vi "Eurotherm - Front Panel.vi"() -> ()   [LabVIEW 2011]
uses:
  Common/Utilities/VI Control/Control - Display State.ctl
panel:
  in  "Setup":bool
  out "Activity":bool
  out "Numeric":i32
  in  "stop":bool
  in  "Tab Control":T1(tab)
  in  "Set Point Read":dbl format="%.3f"
  in  "Ramp Rate 1":dbl format="%.3f"
  in  "Type 1":u16(ring) items=["Step", "Ramp"]
  in  "Clear Graph 1":bool
  in  "AutoTune 1":bool
  out "XY Graph 1":cluster{"Data":cluster{"Time":dbl, "Y":dbl}[]}[](graph)
  out "Temp 1":dbl format="%.3f"
  out "Heater Output 1":dbl format="%.3f"
  in  "Max Output 1":dbl format="%.3f"
  in  "D 1":dbl format="%.3f"
  in  "I 1":dbl format="%.3f"
  in  "P 1":dbl format="%.3f"
  in  "Set Point 1":dbl min=0.0 max=40.0 format="%.3f"
  in  "Set Point Read 2":dbl format="%.3f"
  in  "P 2":dbl format="%.3f"
  in  "I 2":dbl format="%.3f"
  in  "D 2":dbl format="%.3f"
  out "Temp 2":dbl format="%.3f"
  out "Heater Output 2":dbl format="%.3f"
  in  "Set Point 2":dbl min=0.0 max=40.0 format="%.3f"
  in  "Max Output 2":dbl format="%.3f"
  out "XY Graph 2":cluster{"Data":cluster{"Time":dbl, "Y":dbl}[]}[](graph)
  in  "AutoTune 2":bool
  in  "Clear Graph 2":bool
  in  "Type 2":u16(ring) items=["Step", "Ramp"]
  in  "Ramp Rate 2":dbl format="%.3f"
  in  "P 3":dbl format="%.3f"
  in  "I 3":dbl format="%.3f"
  in  "D 3":dbl format="%.3f"
  out "Temp 3":dbl format="%.3f"
  out "Heater Output 3":dbl format="%.3f"
  in  "Set Point 3":dbl min=0.0 max=100.0 format="%.3f"
  in  "Max Output 3":dbl format="%.3f"
  out "XY Graph 3":cluster{"Data":cluster{"Time":dbl, "Y":dbl}[]}[](graph)
  in  "AutoTune 3":bool
  in  "Clear Graph 3":bool
  in  "Type 3":u16(ring) items=["Step", "Ramp"]
  in  "Ramp Rate 3":dbl format="%.3f"
  in  "Set Point Read 3":dbl format="%.3f"
  in  "P 4":dbl format="%.3f"
  in  "I 4":dbl format="%.3f"
  in  "D 4":dbl format="%.3f"
  out "Temp 4":dbl format="%.3f"
  out "Heater Output 4":dbl format="%.3f"
  in  "Set Point 4":dbl min=0.0 max=100.0 format="%.3f"
  in  "Max Output 4":dbl format="%.3f"
  out "XY Graph 4":cluster{"Data":cluster{"Time":dbl, "Y":dbl}[]}[](graph)
  in  "AutoTune 4":bool
  in  "Clear Graph 4":bool
  in  "Type 4":u16(ring) items=["Step", "Ramp"]
  in  "Ramp Rate 4":dbl format="%.3f"
  in  "Set Point Read 4":dbl format="%.3f"
  in  "P 5":dbl format="%.3f"
  in  "I 5":dbl format="%.3f"
  in  "D 5":dbl format="%.3f"
  out "Temp 5":dbl format="%.3f"
  out "Heater Output 5":dbl format="%.3f"
  in  "Set Point 5":dbl min=0.0 max=100.0 format="%.3f"
  in  "Max Output 5":dbl format="%.3f"
  out "XY Graph 5":cluster{"Data":cluster{"Time":dbl, "Y":dbl}[]}[](graph)
  in  "AutoTune 5":bool
  in  "Clear Graph 5":bool
  in  "Type 5":u16(ring) items=["Step", "Ramp"]
  in  "Ramp Rate 5":dbl format="%.3f"
  in  "Set Point Read 5":dbl format="%.3f"
  in  "P 6":dbl format="%.3f"
  in  "I 6":dbl format="%.3f"
  in  "D 6":dbl format="%.3f"
  out "Temp 6":dbl format="%.3f"
  out "Heater Output 6":dbl format="%.3f"
  in  "Set Point 6":dbl min=0.0 max=100.0 format="%.3f"
  in  "Max Output 6":dbl format="%.3f"
  out "XY Graph 6":cluster{"Data":cluster{"Time":dbl, "Y":dbl}[]}[](graph)
  in  "AutoTune 6":bool
  in  "Clear Graph 6":bool
  in  "Type 6":u16(ring) items=["Step", "Ramp"]
  in  "Ramp Rate 6":dbl format="%.3f"
  in  "Set Point Read 6":dbl format="%.3f"
  in  "P 7":dbl format="%.3f"
  in  "I 7":dbl format="%.3f"
  in  "D 7":dbl format="%.3f"
  out "Temp 7":dbl format="%.3f"
  out "Heater Output 7":dbl format="%.3f"
  in  "Set Point 7":dbl min=0.0 max=100.0 format="%.3f"
  in  "Max Output 7":dbl format="%.3f"
  out "XY Graph 7":cluster{"Data":cluster{"Time":dbl, "Y":dbl}[]}[](graph)
  in  "AutoTune 7":bool
  in  "Clear Graph 7":bool
  in  "Type 7":u16(ring) items=["Step", "Ramp"]
  in  "Ramp Rate 7":dbl format="%.3f"
  in  "Set Point Read 7":dbl format="%.3f"
  in  "P 8":dbl format="%.3f"
  in  "I 8":dbl format="%.3f"
  in  "D 8":dbl format="%.3f"
  out "Temp 8":dbl format="%.3f"
  out "Heater Output 8":dbl format="%.3f"
  in  "Set Point 8":dbl min=0.0 max=100.0 format="%.3f"
  in  "Max Output 8":dbl format="%.3f"
  out "XY Graph 8":cluster{"Data":cluster{"Time":dbl, "Y":dbl}[]}[](graph)
  in  "AutoTune 8":bool
  in  "Clear Graph 8":bool
  in  "Type 8":u16(ring) items=["Step", "Ramp"]
  in  "Ramp Rate 8":dbl format="%.3f"
  in  "Set Point Read 8":dbl format="%.3f"
  # "Eurotherm Temperature Controller"
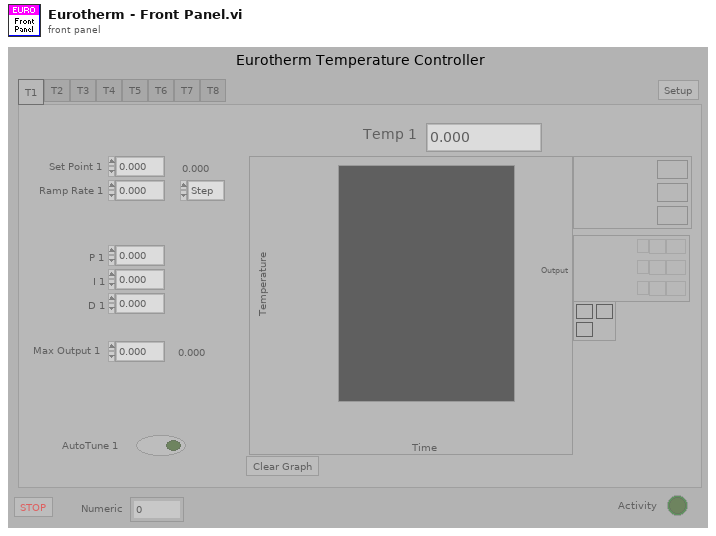
[diagram p1: front panel]
types:
  T1 = enum32{"Page 1", "Page 2", "Page 3", "Page 4", "T5", "T5 2", "T7", "T8"}
  T2 = typedef "Control - Display State.ctl" = enum16{"Enabled", "Disabled", "Disabled and Grayed"}
  T3 = enum32{"Page Enabled", "Page Disabled", "Page Disabled & Grayed"}
  T4 = cluster{"Temp 1":refnum<vi>, "Set Point 1":refnum<vi>, "P 1":refnum<vi>, "I 1":refnum<vi>, "D 1":refnum<vi>, "Heater Output 1":refnum<vi>, "Max Output 1":refnum<vi>, "XY Graph 1":refnum<vi>, "AutoTune 1":refnum<vi>, "Clear Graph 1":refnum<vi>, "Ramp Rate 1":refnum<vi>, "Type 1":refnum<vi>, "Tab Control":refnum<vi>, "Set Point Read":refnum<vi>}
  T5 = cluster{"Temp 2":refnum<vi>, "Set Point 2":refnum<vi>, "P 2":refnum<vi>, "I 2":refnum<vi>, "D 2":refnum<vi>, "Heater Output 2":refnum<vi>, "Max Output 2":refnum<vi>, "XY Graph 2":refnum<vi>, "AutoTune 2":refnum<vi>, "Clear Graph 2":refnum<vi>, "Ramp Rate 2":refnum<vi>, "Type 2":refnum<vi>, "Tab Control":refnum<vi>, "Set Point Read 2":refnum<vi>}
  T6 = cluster{"Temp 3":refnum<vi>, "Set Point 3":refnum<vi>, "P 3":refnum<vi>, "I 3":refnum<vi>, "D 3":refnum<vi>, "Heater Output 3":refnum<vi>, "Max Output 3":refnum<vi>, "XY Graph 3":refnum<vi>, "AutoTune 3":refnum<vi>, "Clear Graph 3":refnum<vi>, "Ramp Rate 3":refnum<vi>, "Type 3":refnum<vi>, "Tab Control":refnum<vi>, "Set Point Read 3":refnum<vi>}
  T7 = cluster{"Temp 4":refnum<vi>, "Set Point 4":refnum<vi>, "P 4":refnum<vi>, "I 4":refnum<vi>, "D 4":refnum<vi>, "Heater Output 4":refnum<vi>, "Max Output 4":refnum<vi>, "XY Graph 4":refnum<vi>, "AutoTune 4":refnum<vi>, "Clear Graph 4":refnum<vi>, "Ramp Rate 4":refnum<vi>, "Type 4":refnum<vi>, "Tab Control":refnum<vi>, "Set Point Read 4":refnum<vi>}
  T8 = cluster{"Temp 5":refnum<vi>, "Set Point 5":refnum<vi>, "P 5":refnum<vi>, "I 5":refnum<vi>, "D 5":refnum<vi>, "Heater Output 5":refnum<vi>, "Max Output 5":refnum<vi>, "XY Graph 5":refnum<vi>, "AutoTune 5":refnum<vi>, "Clear Graph 5":refnum<vi>, "Ramp Rate 5":refnum<vi>, "Type 5":refnum<vi>, "Tab Control":refnum<vi>, "Set Point Read 5":refnum<vi>}
  T9 = cluster{"Temp 6":refnum<vi>, "Set Point 6":refnum<vi>, "P 6":refnum<vi>, "I 6":refnum<vi>, "D 6":refnum<vi>, "Heater Output 6":refnum<vi>, "Max Output 6":refnum<vi>, "XY Graph 6":refnum<vi>, "AutoTune 6":refnum<vi>, "Clear Graph 6":refnum<vi>, "Ramp Rate 6":refnum<vi>, "Type 6":refnum<vi>, "Tab Control":refnum<vi>, "Set Point Read 6":refnum<vi>}
  T10 = cluster{"Temp 7":refnum<vi>, "Set Point 7":refnum<vi>, "P 7":refnum<vi>, "I 7":refnum<vi>, "D 7":refnum<vi>, "Heater Output 7":refnum<vi>, "Max Output 7":refnum<vi>, "XY Graph 7":refnum<vi>, "AutoTune 7":refnum<vi>, "Clear Graph 7":refnum<vi>, "Ramp Rate 7":refnum<vi>, "Type 7":refnum<vi>, "Tab Control":refnum<vi>, "Set Point Read 7":refnum<vi>}
  T11 = cluster{"Temp 8":refnum<vi>, "Set Point 8":refnum<vi>, "P 8":refnum<vi>, "I 8":refnum<vi>, "D 8":refnum<vi>, "Heater Output 8":refnum<vi>, "Max Output 8":refnum<vi>, "XY Graph 8":refnum<vi>, "AutoTune 8":refnum<vi>, "Clear Graph 8":refnum<vi>, "Ramp Rate 8":refnum<vi>, "Type 8":refnum<vi>, "Tab Control":refnum<vi>, "Set Point Read 8":refnum<vi>}
  T12 = typedef "Eurotherm - Setups.ctl" = T13[]
  T13 = typedef "Eurotherm - Setup.ctl" = cluster{"Communication":T14, "Name":string, "Enable":bool, "Max Set Point":dbl, "Min Set Point":dbl, "Units":string, "Graph Data":u32, "Sensor type":T18, "Calibration File Path":path, "Conversion Type":T19}
  T14 = typedef "Eurotherm - Communication.ctl" = cluster{"Com Port":T15, "Address":T16, "Baud Rate":T17}
  T15 = typedef "Com Port - Numeric.ctl" = i32
  T16 = typedef "Eurotherm - Address.ctl" = u8
  T17 = typedef "Com Port - Baud Rate.ctl" = u32
  T18 = typedef "Sensors - Temperature Sensor Type.ctl" = enum16{"RhFe", "Pt", "K type thermocouple", "W5 type thermocouple", "No Conversion"}
  T19 = typedef "Sensors - Conversion Type.ctl" = enum16{"Linear", "Spline"}
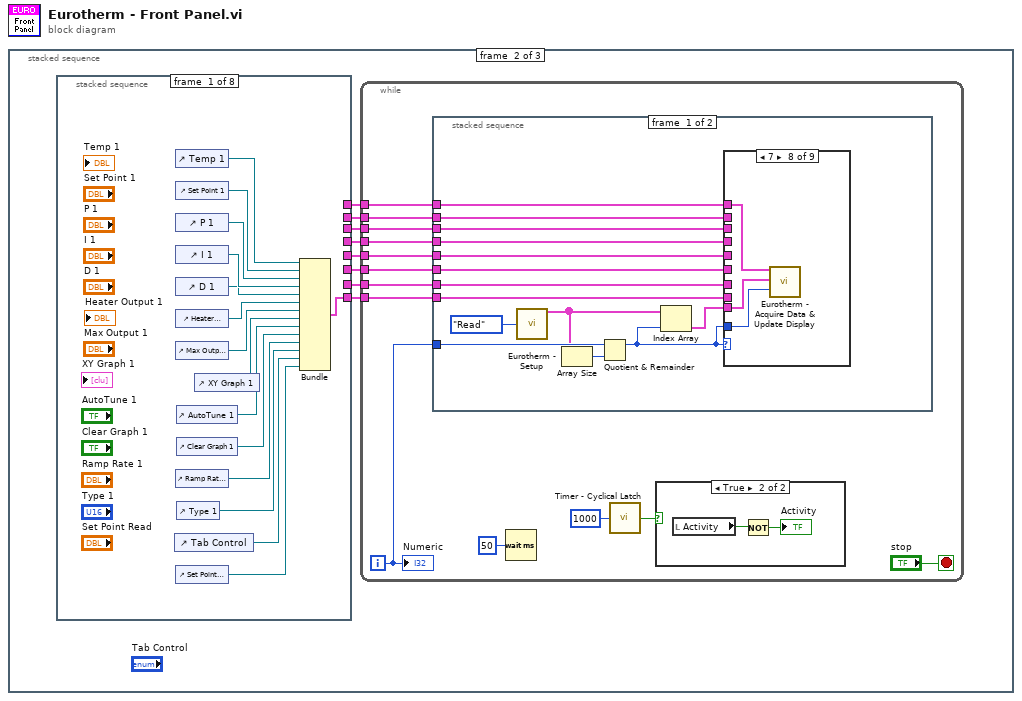
[diagram p0: block diagram]
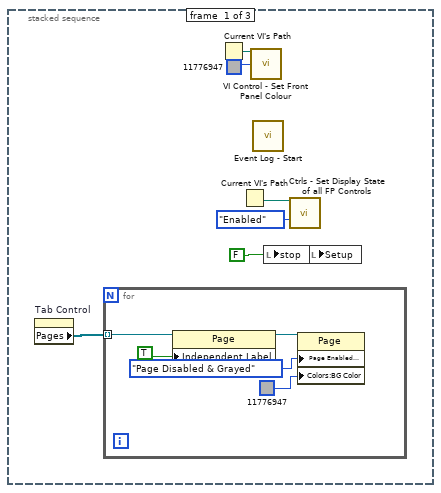
[diagram p2: hidden frame]
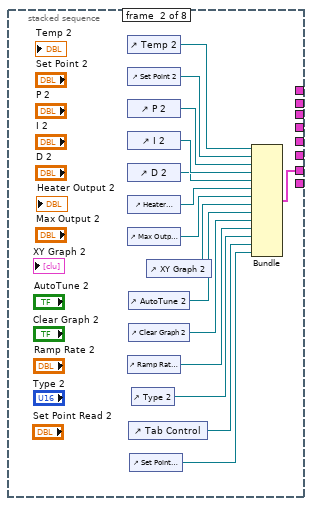
[diagram p3: hidden frame]
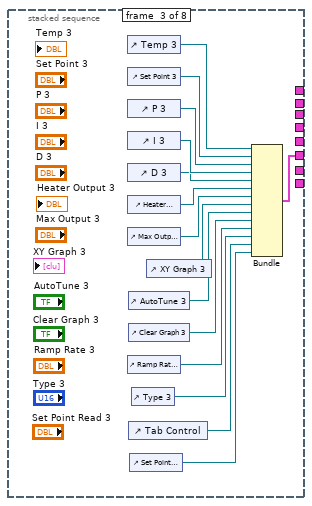
[diagram p4: hidden frame]
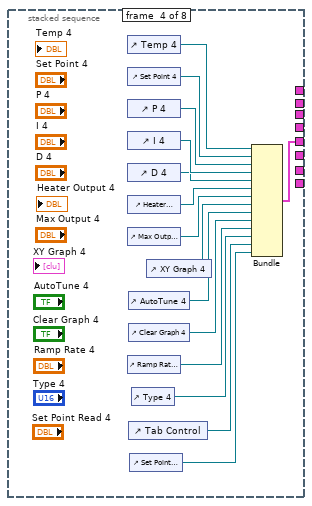
[diagram p5: hidden frame]
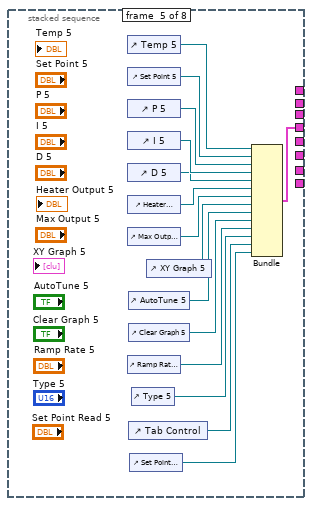
[diagram p6: hidden frame]
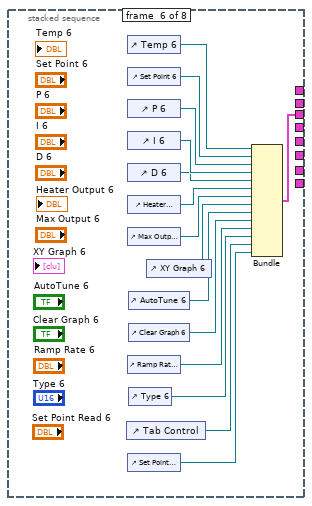
[diagram p7: hidden frame]
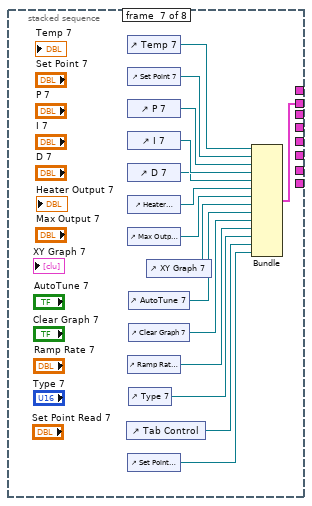
[diagram p8: hidden frame]
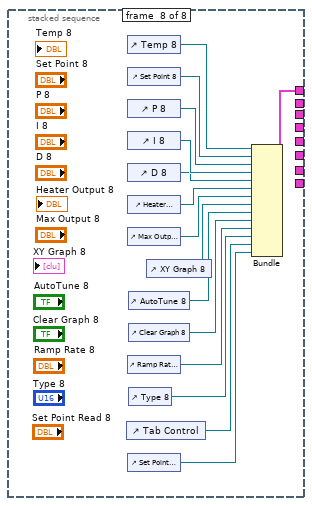
[diagram p9: hidden frame]
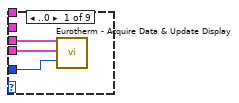
[diagram p10: hidden frame]
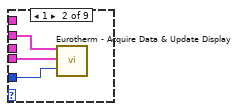
[diagram p11: hidden frame]
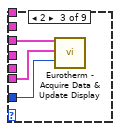
[diagram p12: hidden frame]
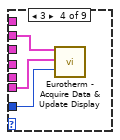
[diagram p13: hidden frame]
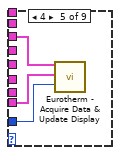
[diagram p14: hidden frame]
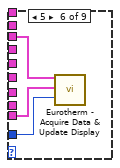
[diagram p15: hidden frame]
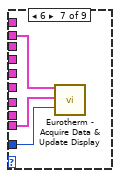
[diagram p16: hidden frame]
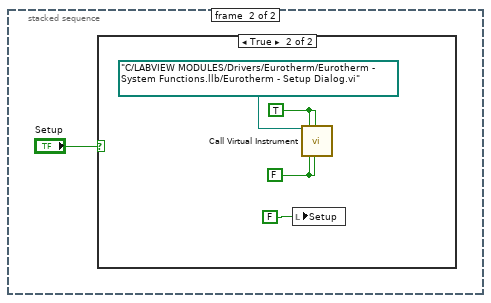
[diagram p18: hidden frame]
diagram:
  n1 = stacked-sequence {
    frame #0 {
      w1 = FALSE
      n2 = property on="Tab Control" class="TabCtl (strict)"() -> ("Pages"=w4:refnum<vi>[])  [unwired: 2 in, 2 out]
      n3 = for {
        tunnel: w4 -> [w9] mode=indexing
        n4 = property class="Page"(reference=w9, "Independent Label"=TRUE) -> (reference out=w10:refnum<vi>)  [unwired: 1 in, 1 out]
        n5 = property class="Page"(reference=w10, "Page Enabled State"=T3."Page Disabled & Grayed", "Colors:BG Color"=u32 11776947) -> ()  [unwired: 1 in, 2 out]
      }
      n6 = Current VI's Path() -> (path=w2:path)
      n7 = Current VI's Path() -> (path=w6:path)
      n8 = call "VI Control - Set Front Panel Colour.vi"("VI Path"=w2, "Front Panel Colour"=u32 11776947) -> ()  [unwired: 13 in, 1 out]
      n9 = call "Event Log - Start.vi"() -> ()  [unwired: 1 in]
      n10 = local write "stop"(w1) -> ()
      n11 = call "Ctrls - Set Display State of all FP Controls.vi"("VI Path"=w6, "Display State"=Control_-_Display_State."Enabled") -> ()  [unwired: 18 in]
      n12 = local write "Setup"(w1) -> ()
    }
    frame #1 {
      n13 = stacked-sequence {
        tunnel: [w26 _ _ _ _ _ _ _] -> w19
        tunnel: [_ w36 _ _ _ _ _ _] -> w18
        tunnel: [_ _ w50 _ _ _ _ _] -> w17
        tunnel: [_ _ _ w65 _ _ _ _] -> w16
        tunnel: [_ _ _ _ w80 _ _ _] -> w15
        tunnel: [_ _ _ _ _ w95 _ _] -> w14
        tunnel: [_ _ _ _ _ _ w110 _] -> w13
        tunnel: [_ _ _ _ _ _ _ w125] -> w12
        frame #0 {
          n14 = control-ref of="Tab Control"() -> (w21:refnum<vi>)
          n15 = control-ref of="Temp 1"() -> (w34:refnum<vi>)
          n16 = control-ref of="Set Point 1"() -> (w33:refnum<vi>)
          n17 = control-ref of="P 1"() -> (w32:refnum<vi>)
          n18 = control-ref of="I 1"() -> (w31:refnum<vi>)
          n19 = control-ref of="D 1"() -> (w30:refnum<vi>)
          n20 = control-ref of="Heater Output 1"() -> (w29:refnum<vi>)
          n21 = control-ref of="Max Output 1"() -> (w28:refnum<vi>)
          n22 = control-ref of="Ramp Rate 1"() -> (w23:refnum<vi>)
          n23 = control-ref of="Set Point Read"() -> (w20:refnum<vi>)
          n24 = control-ref of="AutoTune 1"() -> (w25:refnum<vi>)
          n25 = control-ref of="Clear Graph 1"() -> (w24:refnum<vi>)
          n26 = control-ref of="Type 1"() -> (w22:refnum<vi>)
          n27 = control-ref of="XY Graph 1"() -> (w27:refnum<vi>)
          n28 = Bundle("Temp 1"=w34, "Set Point 1"=w33, "P 1"=w32, "I 1"=w31, "D 1"=w30, "Heater Output 1"=w29, "Max Output 1"=w28, "XY Graph 1"=w27, "AutoTune 1"=w25, "Clear Graph 1"=w24, "Ramp Rate 1"=w23, "Type 1"=w22, "Tab Control"=w21, "Set Point Read"=w20) -> (w26:T4)  [unwired: 1 in]
        }
        frame #1 {
          n29 = control-ref of="Temp 2"() -> (w49:refnum<vi>)
          n30 = control-ref of="Set Point 2"() -> (w48:refnum<vi>)
          n31 = control-ref of="P 2"() -> (w47:refnum<vi>)
          n32 = control-ref of="I 2"() -> (w46:refnum<vi>)
          n33 = control-ref of="D 2"() -> (w45:refnum<vi>)
          n34 = control-ref of="Heater Output 2"() -> (w44:refnum<vi>)
          n35 = control-ref of="Max Output 2"() -> (w43:refnum<vi>)
          n36 = control-ref of="Ramp Rate 2"() -> (w39:refnum<vi>)
          n37 = control-ref of="AutoTune 2"() -> (w41:refnum<vi>)
          n38 = control-ref of="Clear Graph 2"() -> (w40:refnum<vi>)
          n39 = control-ref of="Tab Control"() -> (w37:refnum<vi>)
          n40 = control-ref of="Set Point Read 2"() -> (w35:refnum<vi>)
          n41 = control-ref of="Type 2"() -> (w38:refnum<vi>)
          n42 = control-ref of="XY Graph 2"() -> (w42:refnum<vi>)
          n43 = Bundle("Temp 2"=w49, "Set Point 2"=w48, "P 2"=w47, "I 2"=w46, "D 2"=w45, "Heater Output 2"=w44, "Max Output 2"=w43, "XY Graph 2"=w42, "AutoTune 2"=w41, "Clear Graph 2"=w40, "Ramp Rate 2"=w39, "Type 2"=w38, "Tab Control"=w37, "Set Point Read 2"=w35) -> (w36:T5)  [unwired: 1 in]
        }
        frame #2 {
          n44 = control-ref of="Temp 3"() -> (w64:refnum<vi>)
          n45 = control-ref of="Set Point 3"() -> (w63:refnum<vi>)
          n46 = control-ref of="P 3"() -> (w62:refnum<vi>)
          n47 = control-ref of="I 3"() -> (w61:refnum<vi>)
          n48 = control-ref of="D 3"() -> (w60:refnum<vi>)
          n49 = control-ref of="Heater Output 3"() -> (w59:refnum<vi>)
          n50 = control-ref of="Max Output 3"() -> (w58:refnum<vi>)
          n51 = control-ref of="Ramp Rate 3"() -> (w54:refnum<vi>)
          n52 = control-ref of="AutoTune 3"() -> (w56:refnum<vi>)
          n53 = control-ref of="Clear Graph 3"() -> (w55:refnum<vi>)
          n54 = control-ref of="Tab Control"() -> (w52:refnum<vi>)
          n55 = control-ref of="Set Point Read 3"() -> (w51:refnum<vi>)
          n56 = control-ref of="Type 3"() -> (w53:refnum<vi>)
          n57 = control-ref of="XY Graph 3"() -> (w57:refnum<vi>)
          n58 = Bundle("Temp 3"=w64, "Set Point 3"=w63, "P 3"=w62, "I 3"=w61, "D 3"=w60, "Heater Output 3"=w59, "Max Output 3"=w58, "XY Graph 3"=w57, "AutoTune 3"=w56, "Clear Graph 3"=w55, "Ramp Rate 3"=w54, "Type 3"=w53, "Tab Control"=w52, "Set Point Read 3"=w51) -> (w50:T6)  [unwired: 1 in]
        }
        frame #3 {
          n59 = control-ref of="Temp 4"() -> (w79:refnum<vi>)
          n60 = control-ref of="Set Point 4"() -> (w78:refnum<vi>)
          n61 = control-ref of="P 4"() -> (w77:refnum<vi>)
          n62 = control-ref of="I 4"() -> (w76:refnum<vi>)
          n63 = control-ref of="D 4"() -> (w75:refnum<vi>)
          n64 = control-ref of="Heater Output 4"() -> (w74:refnum<vi>)
          n65 = control-ref of="Max Output 4"() -> (w73:refnum<vi>)
          n66 = control-ref of="Ramp Rate 4"() -> (w69:refnum<vi>)
          n67 = control-ref of="AutoTune 4"() -> (w71:refnum<vi>)
          n68 = control-ref of="Clear Graph 4"() -> (w70:refnum<vi>)
          n69 = control-ref of="Tab Control"() -> (w67:refnum<vi>)
          n70 = control-ref of="Set Point Read 4"() -> (w66:refnum<vi>)
          n71 = control-ref of="Type 4"() -> (w68:refnum<vi>)
          n72 = control-ref of="XY Graph 4"() -> (w72:refnum<vi>)
          n73 = Bundle("Temp 4"=w79, "Set Point 4"=w78, "P 4"=w77, "I 4"=w76, "D 4"=w75, "Heater Output 4"=w74, "Max Output 4"=w73, "XY Graph 4"=w72, "AutoTune 4"=w71, "Clear Graph 4"=w70, "Ramp Rate 4"=w69, "Type 4"=w68, "Tab Control"=w67, "Set Point Read 4"=w66) -> (w65:T7)  [unwired: 1 in]
        }
        frame #4 {
          n74 = control-ref of="Temp 5"() -> (w94:refnum<vi>)
          n75 = control-ref of="Set Point 5"() -> (w93:refnum<vi>)
          n76 = control-ref of="P 5"() -> (w92:refnum<vi>)
          n77 = control-ref of="I 5"() -> (w91:refnum<vi>)
          n78 = control-ref of="D 5"() -> (w90:refnum<vi>)
          n79 = control-ref of="Heater Output 5"() -> (w89:refnum<vi>)
          n80 = control-ref of="Max Output 5"() -> (w88:refnum<vi>)
          n81 = control-ref of="Ramp Rate 5"() -> (w84:refnum<vi>)
          n82 = control-ref of="AutoTune 5"() -> (w86:refnum<vi>)
          n83 = control-ref of="Clear Graph 5"() -> (w85:refnum<vi>)
          n84 = control-ref of="Tab Control"() -> (w82:refnum<vi>)
          n85 = control-ref of="Set Point Read 5"() -> (w81:refnum<vi>)
          n86 = control-ref of="Type 5"() -> (w83:refnum<vi>)
          n87 = control-ref of="XY Graph 5"() -> (w87:refnum<vi>)
          n88 = Bundle("Temp 5"=w94, "Set Point 5"=w93, "P 5"=w92, "I 5"=w91, "D 5"=w90, "Heater Output 5"=w89, "Max Output 5"=w88, "XY Graph 5"=w87, "AutoTune 5"=w86, "Clear Graph 5"=w85, "Ramp Rate 5"=w84, "Type 5"=w83, "Tab Control"=w82, "Set Point Read 5"=w81) -> (w80:T8)  [unwired: 1 in]
        }
        frame #5 {
          n89 = control-ref of="Tab Control"() -> (w97:refnum<vi>)
          n90 = control-ref of="Temp 6"() -> (w109:refnum<vi>)
          n91 = control-ref of="Set Point 6"() -> (w108:refnum<vi>)
          n92 = control-ref of="P 6"() -> (w107:refnum<vi>)
          n93 = control-ref of="I 6"() -> (w106:refnum<vi>)
          n94 = control-ref of="D 6"() -> (w105:refnum<vi>)
          n95 = control-ref of="Heater Output 6"() -> (w104:refnum<vi>)
          n96 = control-ref of="Max Output 6"() -> (w103:refnum<vi>)
          n97 = control-ref of="Ramp Rate 6"() -> (w99:refnum<vi>)
          n98 = control-ref of="Set Point Read 6"() -> (w96:refnum<vi>)
          n99 = control-ref of="AutoTune 6"() -> (w101:refnum<vi>)
          n100 = control-ref of="Clear Graph 6"() -> (w100:refnum<vi>)
          n101 = control-ref of="Type 6"() -> (w98:refnum<vi>)
          n102 = control-ref of="XY Graph 6"() -> (w102:refnum<vi>)
          n103 = Bundle("Temp 6"=w109, "Set Point 6"=w108, "P 6"=w107, "I 6"=w106, "D 6"=w105, "Heater Output 6"=w104, "Max Output 6"=w103, "XY Graph 6"=w102, "AutoTune 6"=w101, "Clear Graph 6"=w100, "Ramp Rate 6"=w99, "Type 6"=w98, "Tab Control"=w97, "Set Point Read 6"=w96) -> (w95:T9)  [unwired: 1 in]
        }
        frame #6 {
          n104 = control-ref of="Tab Control"() -> (w112:refnum<vi>)
          n105 = control-ref of="Temp 7"() -> (w124:refnum<vi>)
          n106 = control-ref of="Set Point 7"() -> (w123:refnum<vi>)
          n107 = control-ref of="P 7"() -> (w122:refnum<vi>)
          n108 = control-ref of="I 7"() -> (w121:refnum<vi>)
          n109 = control-ref of="D 7"() -> (w120:refnum<vi>)
          n110 = control-ref of="Heater Output 7"() -> (w119:refnum<vi>)
          n111 = control-ref of="Max Output 7"() -> (w118:refnum<vi>)
          n112 = control-ref of="Ramp Rate 7"() -> (w114:refnum<vi>)
          n113 = control-ref of="Set Point Read 7"() -> (w111:refnum<vi>)
          n114 = control-ref of="AutoTune 7"() -> (w116:refnum<vi>)
          n115 = control-ref of="Clear Graph 7"() -> (w115:refnum<vi>)
          n116 = control-ref of="Type 7"() -> (w113:refnum<vi>)
          n117 = control-ref of="XY Graph 7"() -> (w117:refnum<vi>)
          n118 = Bundle("Temp 7"=w124, "Set Point 7"=w123, "P 7"=w122, "I 7"=w121, "D 7"=w120, "Heater Output 7"=w119, "Max Output 7"=w118, "XY Graph 7"=w117, "AutoTune 7"=w116, "Clear Graph 7"=w115, "Ramp Rate 7"=w114, "Type 7"=w113, "Tab Control"=w112, "Set Point Read 7"=w111) -> (w110:T10)  [unwired: 1 in]
        }
        frame #7 {
          n119 = control-ref of="Tab Control"() -> (w127:refnum<vi>)
          n120 = control-ref of="Temp 8"() -> (w139:refnum<vi>)
          n121 = control-ref of="Set Point 8"() -> (w138:refnum<vi>)
          n122 = control-ref of="P 8"() -> (w137:refnum<vi>)
          n123 = control-ref of="I 8"() -> (w136:refnum<vi>)
          n124 = control-ref of="D 8"() -> (w135:refnum<vi>)
          n125 = control-ref of="Heater Output 8"() -> (w134:refnum<vi>)
          n126 = control-ref of="Max Output 8"() -> (w133:refnum<vi>)
          n127 = control-ref of="Ramp Rate 8"() -> (w129:refnum<vi>)
          n128 = control-ref of="Set Point Read 8"() -> (w126:refnum<vi>)
          n129 = control-ref of="AutoTune 8"() -> (w131:refnum<vi>)
          n130 = control-ref of="Clear Graph 8"() -> (w130:refnum<vi>)
          n131 = control-ref of="Type 8"() -> (w128:refnum<vi>)
          n132 = control-ref of="XY Graph 8"() -> (w132:refnum<vi>)
          n133 = Bundle("Temp 8"=w139, "Set Point 8"=w138, "P 8"=w137, "I 8"=w136, "D 8"=w135, "Heater Output 8"=w134, "Max Output 8"=w133, "XY Graph 8"=w132, "AutoTune 8"=w131, "Clear Graph 8"=w130, "Ramp Rate 8"=w129, "Type 8"=w128, "Tab Control"=w127, "Set Point Read 8"=w126) -> (w125:T11)  [unwired: 1 in]
        }
      }
      n134 = while {
        tunnel: w19 -> [w151]
        tunnel: w18 -> [w148]
        tunnel: w17 -> [w147]
        tunnel: w16 -> [w144]
        tunnel: w15 -> [w143]
        tunnel: w14 -> [w142]
        tunnel: w13 -> [w141]
        tunnel: w12 -> [w140]
        i -> [w150]
        stop <- "stop" stop-if-true
        n135 = stacked-sequence {
          tunnel: w151 -> [w166 _]
          tunnel: w150 -> [w165 _]
          tunnel: w148 -> [w160 _]
          tunnel: w147 -> [w158 _]
          tunnel: w144 -> [w157 _]
          tunnel: w143 -> [w156 _]
          tunnel: w142 -> [w155 _]
          tunnel: w141 -> [w154 _]
          tunnel: w140 -> [w153 _]
          frame #0 {
            n136 = call "Eurotherm - Setup.vi"("Action"=enum16{"Read", "Write"}."Read") -> ("Setup Out"=w162:T12)  [unwired: 12 in, 2 out]
            n137 = Array Size(array=w162) -> (size(s)=w163:i32)
            n138 = Quotient & Remainder(x=w165, y=w163) -> (x-y*floor(x/y)=w159:i32)  [unwired: 1 out]
            n139 = Index Array(array=w162, index=w159) -> (element=w161:T13)
            n140 = case shown="7" w159 {
              tunnel: w166 -> [w168 _ _ _ _ _ _ _ _]
              tunnel: w161 -> [w169 w172 w174 w177 w180 w183 w186 w189 _]
              tunnel: w160 -> [_ w170 _ _ _ _ _ _ _]
              tunnel: w159 -> [w167 w171 w175 w178 w181 w184 w187 w190 _]
              tunnel: w158 -> [_ _ w173 _ _ _ _ _ _]
              tunnel: w157 -> [_ _ _ w176 _ _ _ _ _]
              tunnel: w156 -> [_ _ _ _ w179 _ _ _ _]
              tunnel: w155 -> [_ _ _ _ _ w182 _ _ _]
              tunnel: w154 -> [_ _ _ _ _ _ w185 _ _]
              tunnel: w153 -> [_ _ _ _ _ _ _ w188 _]
              frame ..0 {
                n141 = call "Eurotherm - Acquire Data & Update Display.vi"("Control References"=w168, "Eurotherm Setup"=w169, "Index"=w167) -> ()  [unwired: 17 in]
              }
              frame 1 {
                n142 = call "Eurotherm - Acquire Data & Update Display.vi"("Control References"=w170, "Eurotherm Setup"=w172, "Index"=w171) -> ()  [unwired: 17 in]
              }
              frame 2 {
                n143 = call "Eurotherm - Acquire Data & Update Display.vi"("Control References"=w173, "Eurotherm Setup"=w174, "Index"=w175) -> ()  [unwired: 17 in]
              }
              frame 3 {
                n144 = call "Eurotherm - Acquire Data & Update Display.vi"("Control References"=w176, "Eurotherm Setup"=w177, "Index"=w178) -> ()  [unwired: 17 in]
              }
              frame 4 {
                n145 = call "Eurotherm - Acquire Data & Update Display.vi"("Control References"=w179, "Eurotherm Setup"=w180, "Index"=w181) -> ()  [unwired: 17 in]
              }
              frame 5 {
                n146 = call "Eurotherm - Acquire Data & Update Display.vi"("Control References"=w182, "Eurotherm Setup"=w183, "Index"=w184) -> ()  [unwired: 17 in]
              }
              frame 6 {
                n147 = call "Eurotherm - Acquire Data & Update Display.vi"("Control References"=w185, "Eurotherm Setup"=w186, "Index"=w187) -> ()  [unwired: 17 in]
              }
              frame 7 {
                n148 = call "Eurotherm - Acquire Data & Update Display.vi"("Control References"=w188, "Eurotherm Setup"=w189, "Index"=w190) -> ()  [unwired: 17 in]
              }
              frame Default {
              }
            }
          }
          frame #1 {
            n149 = case shown="True" "Setup" {
              frame False {
              }
              frame True {
                w193 = FALSE
                w195 = TRUE
                n150 = local write "Setup"(FALSE) -> ()
                n151 = call "Call Virtual Instrument.vi"("Vi Call Location"=path "C:/LABVIEW MODULES/Drivers/Eurotherm/Eurotherm - System Functions.llb/Eurotherm - Setup Dialog.vi", "Open Front Panel Window"=w195, "Wait for end of Execucion"=w193, "Run Vi"=w195, "Close Panel when Finished"=w193) -> ()  [unwired: 14 in, 1 out]
              }
            }
          }
        }
        n152 = Wait (ms)(milliseconds to wait=u32 50) -> ()  [unwired: 1 out]
        n153 = call "Timer - Cyclical Latch.vi"("Timer (msec)"=u32 1000) -> ("Timer Trigger"=w145:bool)  [unwired: 14 in]
        n154 = case shown="True" w145 {
          frame False {
          }
          frame True {
            n155 = local read "Activity"() -> (w196:bool)
            n156 = Not(x=w196) -> (.not. x?=→"Activity":bool)
          }
        }
        "Numeric" <- w150
      }
    }
    frame #2 {
      w198 = FALSE
      n157 = property on="Tab Control" class="TabCtl (strict)"() -> ("Pages"=w201:refnum<vi>[])  [unwired: 2 in, 2 out]
      n158 = for {
        tunnel: w201 -> [w206] mode=indexing
        n159 = property class="Page"(reference=w206, "Independent Label"=TRUE) -> (reference out=w207:refnum<vi>)  [unwired: 1 in, 1 out]
        n160 = property class="Page"(reference=w207, "Page Enabled State"=T3."Page Disabled & Grayed", "Colors:BG Color"=u32 11776947) -> ()  [unwired: 1 in, 2 out]
      }
      n161 = Current VI's Path() -> (path=w199:path)
      n162 = Current VI's Path() -> (path=w203:path)
      n163 = call "Event Log - Finished.vi"() -> ()  [unwired: 1 in]
      n164 = call "VI Control - Set Front Panel Colour.vi"("VI Path"=w199, "Front Panel Colour"=u32 11776947) -> ()  [unwired: 13 in, 1 out]
      n165 = local write "stop"(w198) -> ()
      n166 = call "Ctrls - Set Display State of all FP Controls.vi"("VI Path"=w203, "Display State"=Control_-_Display_State."Disabled and Grayed") -> ()  [unwired: 18 in]
      n167 = local write "Setup"(w198) -> ()
    }
  }
